vi "Find Re-entrant VIs in Folder.vi"(8 "error in (no error)":errorcluster, 10 "Pattern":string[](array[string])=["*.vi"], 11 "Directory Path":path) -> (0 "error out":errorcluster, 3 "VI List":path[](array[path]))   [LabVIEW 2014, in "SLL Application.lvlib"]
doc: "This VI can be used to find the list of broken VIs in a folder. This also returns VIs which are of higher LabVIEW version than the currently used LabVIEW version."
uses:
  SLL Application.lvlib
panel:
  out "Progress":i32
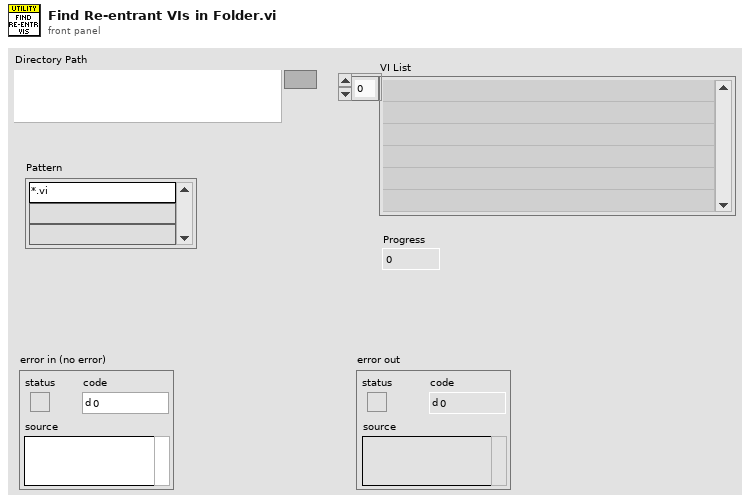
[diagram p1: front panel]
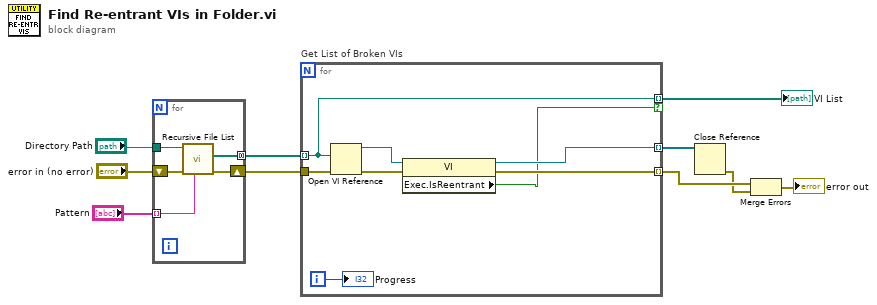
[diagram p0: block diagram]
diagram:
  n1 = for {
    tunnel: "Directory Path" -> [w15]
    tunnel: [w14] -> w8 mode=concatenating
    shift-right: [w12] -> w5
    shift-left: "error in (no error)" -> [w13]
    tunnel: "Pattern" -> [w11] mode=indexing
    n2 = call <vilib>:"Recursive File List.vi"("pattern"=w11, "error in (no error)"=w13, "Folder Path"=w15) -> ("error out"=w12:errorcluster, "All Files in Dir"=w14:path[])  [unwired: 4 in, 3 out]
  }
  n3 = for "Get List of Broken VIs" {
    tunnel: [w22] -> w10 mode=indexing
    tunnel: w8 -> [w21] mode=indexing
    tunnel: [w21] -> w7 mode=indexing if=w16
    tunnel: w5 -> [w20]
    tunnel: [w18] -> w4 mode=indexing
    i -> [w17]
    n4 = Open VI Reference(vi path=w21, error in (no error)=w20) -> (vi reference=w23:refnum<vi>, error out=w19:errorcluster)  [unwired: 4 in]
    n5 = property class="VI"(reference=w23, error in=w19) -> (reference out=w22:refnum<vi>, error out=w18:errorcluster, "Exec.IsReentrant"=w16:bool)
    "Progress" <- w17
  }
  "VI List" <- w7
  n6 = Close Reference(reference=w10) -> (error out=w3:errorcluster)  [unwired: 1 in]
  n7 = Merge Errors(w4, w3) -> (→"error out":errorcluster)
